vi "SUB_READ_Telnet.vi"(3 "timeout ms":i32=25000, 5 "telnet connection":T1) -> (1 "data out":string, 2 "telnet connection out":T1)   [LabVIEW 2011]
uses:
  <vilib>/addons/internet/telnet/telnet.llb/Telnet Session.ctl
  <vilib>/addons/internet/NI_InternetTK_Core_VIs.lvlib
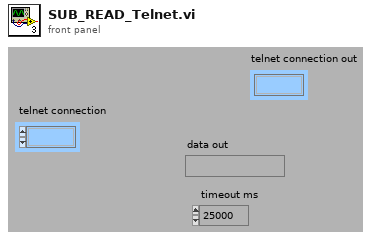
[diagram p1: front panel]
types:
  T1 = typedef "Telnet Session.ctl" = refnum<k1>
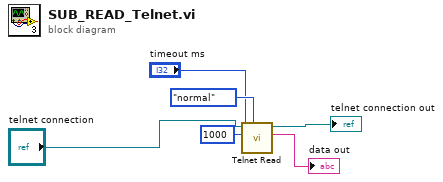
[diagram p0: block diagram]
diagram:
  n1 = call <vilib>:"Telnet Read.vi"("read mode (normal)"=enum16{"normal", "line", "buffered"}."normal", "timeout ms (25000)"="timeout ms", "bytes to read"=1000, "telnet connection"="telnet connection") -> ("data out"=→"data out":string, "telnet connection out"=→"telnet connection out":T1)  [unwired: 3 in, 1 out]
